vi "CreateVirtualFolders.vi"(8 "error in (no error)":errorcluster, 10 "Name":string, 11 "LabVIEW Class In":refnum<vi>) -> (0 "error out":errorcluster, 3 "LabVIEW Class Out":refnum<vi>)   [LabVIEW 2013, in "baseClass.lvclass"]
uses:
  baseClass.lvclass
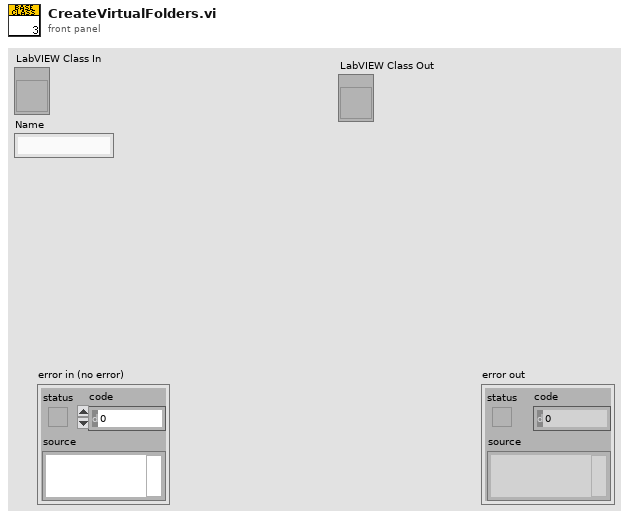
[diagram p1: front panel]
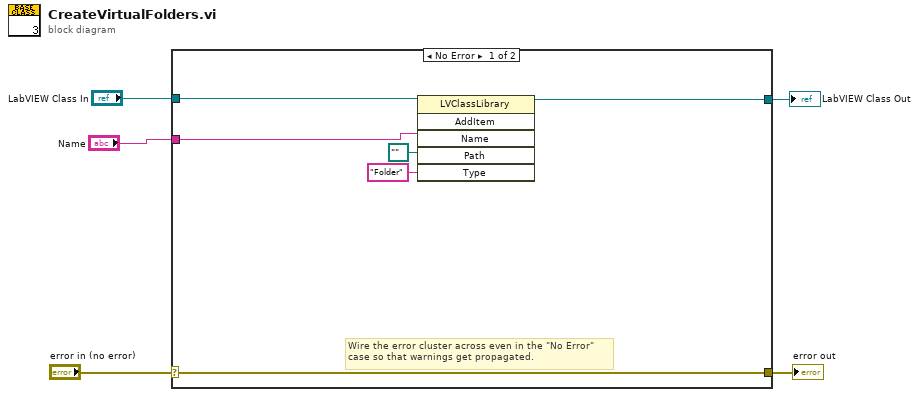
[diagram p0: block diagram]
diagram:
  n1 = case shown="No Error" "error in (no error)" {
    selector: "error in (no error)" -> [w11 w13]
    tunnel: [w11 w13] -> w4
    tunnel: "LabVIEW Class In" -> [w10 w12]
    tunnel: [w9 w12] -> w2
    tunnel: "Name" -> [w6 _]
    frame No Error {
      # "Wire the error cluster across even in the \"No Error\"\ncase so that warnings get propagated."
      n2 = invoke class="LVClassLibrary" method="AddItem"(reference=w10, "Name"=w6, "Path"=path "", "Type"="Folder") -> (reference out=w9:refnum<vi>)  [unwired: 2 in, 5 out]
    }
    frame Error {
    }
  }
  "error out" <- w4
  "LabVIEW Class Out" <- w2
